vi "Spam - Check Spam Duration Elapsed.vi"(8 "Error In":errorcluster, 9 "Spam Started Timestamp":timestamp, 10 "n (ms)":u32=5000 min=100 max=60000 step=100, 11 "Spam Mode":T1) -> (0 "Error Out":errorcluster, 3 "T = Spam duration has elapsed. Need to stop spamming.":bool)   [LabVIEW 2016, in "Anti-Spam Tester (AST).lvlib"]
doc: "Blank VI with error handling."
uses:
  Anti-Spam Tester (AST).lvlib
  Spam Mode (enum).ctl
panel:
  # "Input\nInputs to the VI"
  # "Development\nControls or indicators that are useful for development or testing, but which are not outputs of the VI."
  # "Output\nOutputs of the VI"
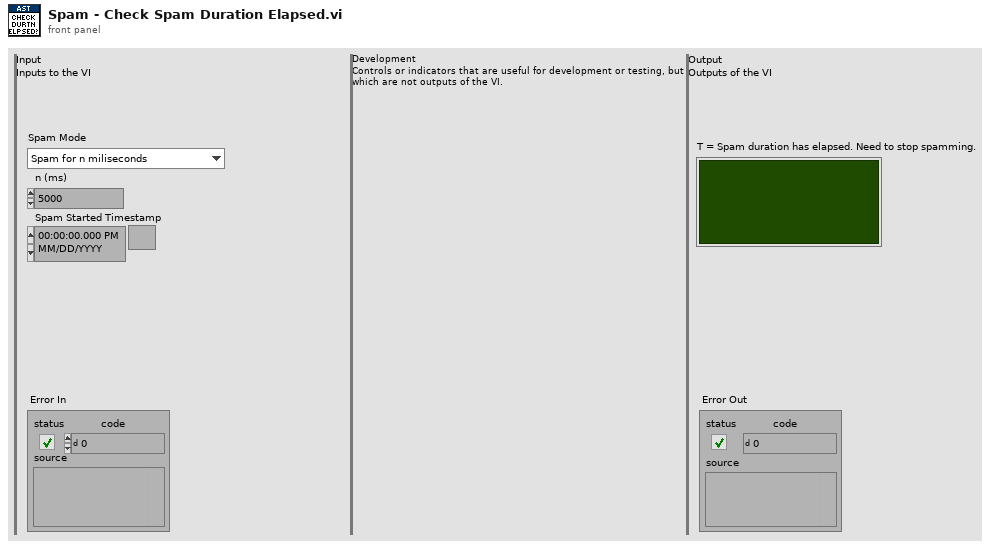
[diagram p1: front panel]
types:
  T1 = typedef "Anti-Spam Tester (AST).lvlib/Spam Mode (enum).ctl" = enum16{"Spam for n miliseconds", "Spam continuously"}
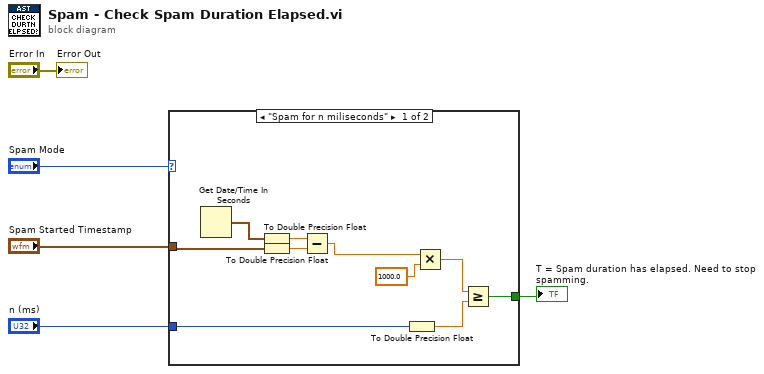
[diagram p0: block diagram]
diagram:
  n1 = case shown="\"Spam for n miliseconds\"" "Spam Mode" {
    tunnel: "Spam Started Timestamp" -> [w14 _]
    tunnel: "n (ms)" -> [w8 _]
    tunnel: [w6 _] -> w1
    frame "Spam for n miliseconds" {
      n2 = Get Date/Time In Seconds() -> (seconds since 1Jan1904=w15:timestamp)
      n3 = To Double Precision Float(number=w15) -> (double precision float=w13:dbl)
      n4 = To Double Precision Float(number=w14) -> (double precision float=w12:dbl)
      n5 = Subtract(x=w13, y=w12) -> (x-y=w11:dbl)
      n6 = To Double Precision Float(number=w8) -> (double precision float=w7:dbl)
      n7 = Multiply(x=w11, y=1000.0) -> (x*y=w9:dbl)
      n8 = Greater Or Equal?(x=w9, y=w7) -> (x >= y?=w6:bool)
    }
    frame "Spam continuously" {
    }
  }
  "T = Spam duration has elapsed. Need to stop spamming." <- w1
  "Error Out" <- "Error In"
